vi "set_config_cluster.vi"(8 "error in (no error)":errorcluster, 10 "config cluster variant":variant, 11 "TrajectoryDL110413StraightLine in":refnum<class "TrajectoryDL110413StraightLine.lvclass">) -> (0 "error out":errorcluster, 3 "TrajectoryDL110413StraightLine out":refnum<class "TrajectoryDL110413StraightLine.lvclass">)   [LabVIEW 2010, in "TrajectoryDL110413StraightLine.lvclass"]
uses:
  TrajectoryDL110413StraightLine.lvclass
  TrajectoryDL110413StraightLine.lvclass/TrajectoryDL110413StraightLine.ctl
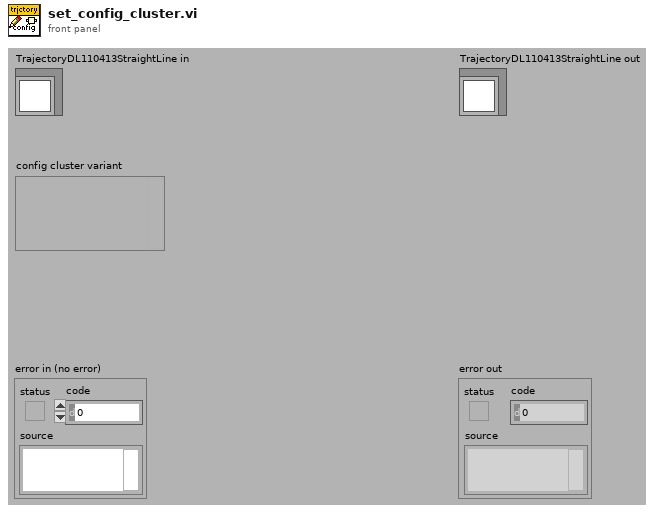
[diagram p1: front panel]
types:
  T1 = typedef "TrajectoryDL110413StraightLine.lvclass/config_data_cluster.ctl" = cluster{"xpaths":cluster{"x offset":string, "y offset":string, "z offset":string}}
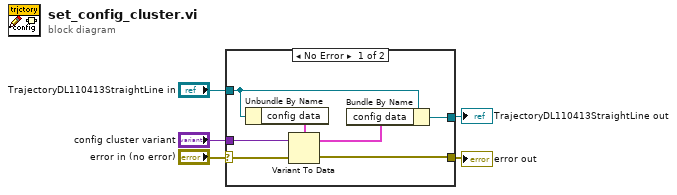
[diagram p0: block diagram]
diagram:
  n1 = case shown="No Error" "error in (no error)" {
    selector: "error in (no error)" -> [w12 w14]
    tunnel: [w7 w14] -> w4
    tunnel: [w6 w13] -> w2
    tunnel: "TrajectoryDL110413StraightLine in" -> [w8 w13]
    tunnel: "config cluster variant" -> [w10 _]
    frame No Error {
      n2 = Unbundle By Name(w8) -> ("config data"=w11:T1)
      n3 = Variant To Data(error in=w12, Variant=w10, type=w11) -> (error out=w7:errorcluster, data=w9:T1)
      n4 = Bundle By Name(cluster=w8, "config data"=w9) -> (w6:refnum<class "TrajectoryDL110413StraightLine.lvclass">)
    }
    frame Error {
    }
  }
  "error out" <- w4
  "TrajectoryDL110413StraightLine out" <- w2
